vi "Serialize.vi"(8 "error in (no error)":errorcluster, 11 "Run VI in":refnum<class "Run VI.lvclass">=refnum) -> (0 "error out":errorcluster, 2 "Text":string)   [LabVIEW 2014, in "Run VI.lvclass"]
uses:
  Run VI.lvclass
  Shared/Controls/Run VI - STYP.ctl
  Classes/Job/Job.lvclass/Job.ctl
  Run VI.lvclass/Run VI.ctl
  Classes/Job/Read Executor Number.vi
  Read VI Path.vi
  Read Wait Until Done_.vi
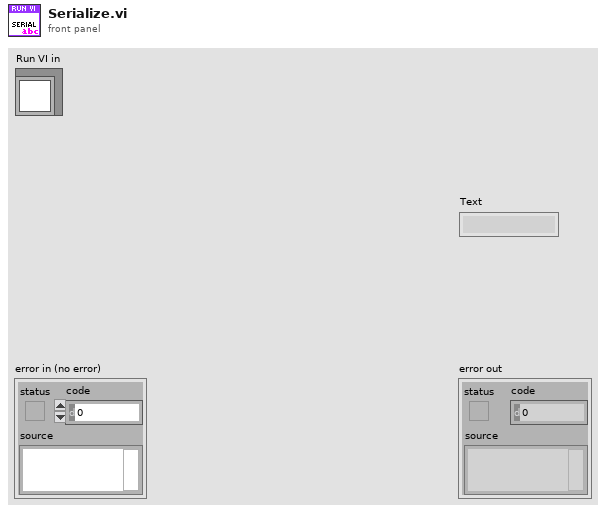
[diagram p1: front panel]
types:
  T1 = typedef "Run VI - STYP.ctl" = cluster{"Executor_Number":string, "VI_Path":string, "Wait_Until_Done":bool}
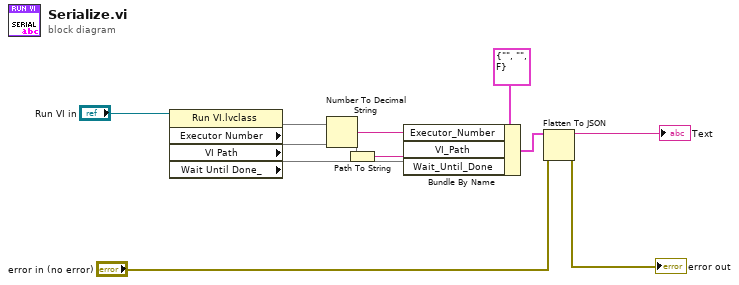
[diagram p0: block diagram]
diagram:
  n1 = property class="Run VI.lvclass"(reference="Run VI in") -> ("Executor Number"=w10, "VI Path"=w4, "Wait Until Done_"=w5)  [unwired: 1 in, 2 out]
  n2 = Number To Decimal String(number=w10) -> (decimal integer string=w6:string)  [unwired: 1 in]
  n3 = Path To String(path=w4) -> (string=w3:string)
  n4 = Bundle By Name(cluster=T1 {"Executor_Number"="", "VI_Path"="", "Wait_Until_Done"=FALSE} ("Run VI"), "Executor_Number"=w6, "VI_Path"=w3, "Wait_Until_Done"=w5) -> (w7:T1)
  n5 = Flatten To JSON(anything=w7, error in (no error)="error in (no error)") -> (JSON string=→"Text":string, 11:→"error out":errorcluster)  [unwired: 1 in]
